vi "Constants.vi"() -> ()   [LabVIEW 2018]
panel:
  in  "ArmDegreesPerSensorUnit":dbl=0.736
  in  "ArmAngle(Horizontal)":dbl=-55.0
  in  "ArmLength":dbl=48.4
  in  "ArmRotatePointHeight":dbl=40.5
  in  "ElevatorSetpoints":dbl[](array[numeric])=[19.0, 47.0, 75.0, 27.5, 55.5, 83.5, 40.0, 0.0, 27.5, 0.0]
  in  "Track Width":dbl=28.0
  in  "CenterRotOffset":dbl=17.0
  in  "Length":dbl=38.5
  in  "Width":dbl=31.5
  # "Make sure to set values as defaults when done!"
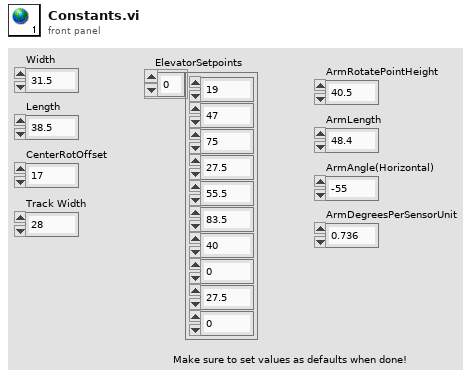
[diagram p1: front panel]
diagram:
